vi "Configure Sensor Break.vi"(0 "VISA resource name":refnum<visa-resource-name>, 1 "Unit Address (1)":u8=1 min=1 max=254, 9 "Sensor Break Type (1: ON)":i16(ring)=1 items=["OFF", "ON", "LAT"], 11 "error in (no error)":errorcluster, 12 "Override Sensor Break (False: Disable)":bool) -> (4 "VISA resource name out":refnum<visa-resource-name>, 15 "error out":errorcluster)   [LabVIEW 2010, in "Eurotherm 32xx Series.lvlib"]
doc: "This VI configures Sensor Break Type.\n\nWarning: This VI uses Controller Configuration Mode, this interrupts working process (device will not control).\nIt is recommended that the device should be disconnected from any active process."
uses:
  <instrlib>/Eurotherm 32xx Series/Eurotherm 32xx Series.lvlib
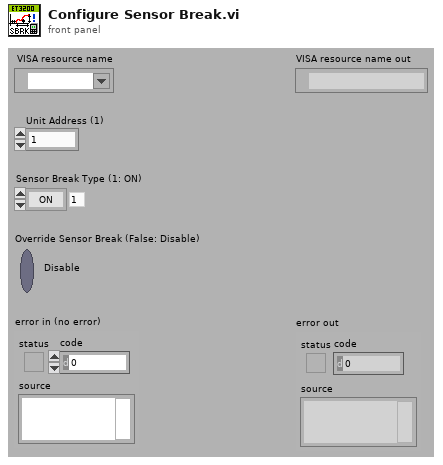
[diagram p1: front panel]
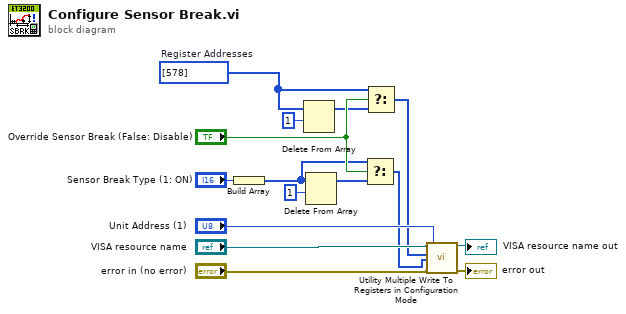
[diagram p0: block diagram]
diagram:
  w11 = u16[] [578]  # Register Addresses
  n1 = Build Array("Sensor Break Type (1: ON)") -> (w9:i16[])
  n2 = Delete From Array(array=w11, length=u16 1) -> (array with subset deleted=w10:u16[])  [unwired: 1 in, 1 out]
  n3 = Delete From Array(array=w9, length=u16 1) -> (array with subset deleted=w8:i16[])  [unwired: 1 in, 1 out]
  n4 = Select(t=w9, s="Override Sensor Break (False: Disable)", f=w8) -> (s? t:f=w4:i16[])
  n5 = Select(t=w11, s="Override Sensor Break (False: Disable)", f=w10) -> (s? t:f=w5:u16[])
  n6 = call <instrlib>:"Utility Multiple Write To Registers in Configuration Mode.vi"("VISA resource name"="VISA resource name", "Unit Address (1)"="Unit Address (1)", "Registers Addresses (0)"=w5, "Data (0)"=w4, "error in (no error)"="error in (no error)") -> ("VISA resource name out"=→"VISA resource name out":refnum<visa-resource-name>, "error out"=→"error out":errorcluster)  [unwired: 9 in]
